vi "test_udp_write.vi"() -> ()   [LabVIEW 2019]
uses:
  <vilib>/Utility/tcp.llb/UDP Multicast Write-Only Open.vi
panel:
  in  "stop":bool
  out "error out":errorcluster
  in  "TopUDPPort":u16=17308
  in  "TopTCPPort":u16=17309
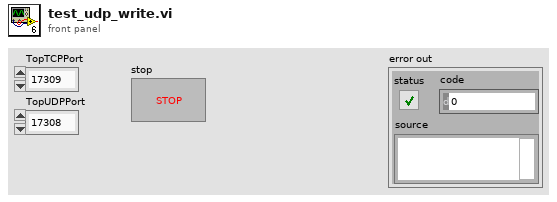
[diagram p1: front panel]
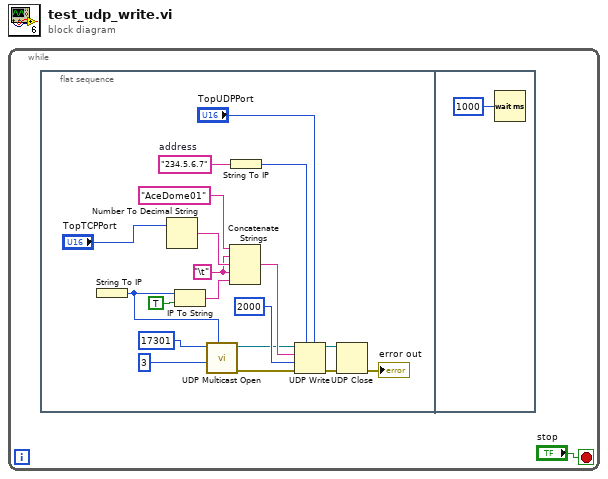
[diagram p0: block diagram]
diagram:
  n1 = while {
    stop <- "stop" stop-if-true
    n2 = flat-sequence {
      frame #0 {
        w13 = "\t"
        w18 = "234.5.6.7"  # address
        n3 = String To IP() -> (0:w6:u32)  [unwired: 1 in]
        n4 = Number To Decimal String(number="TopTCPPort") -> (decimal integer string=w15:string)  [unwired: 1 in]
        n5 = IP To String(1:TRUE ("dot notation? (F)"), 2:w6) -> (0:w11:string)
        n6 = call-poly <vilib>:"UDP Multicast Open.vi"("net address"=w6, "time-to-live (1)"=u16 3, "port"=u16 17301) -> ("error out"=w7:errorcluster, "connection ID"=w8:refnum<k16>)  [unwired: 7 in]
        n7 = Concatenate Strings("AceDome01" ("string"), w13, w15, w13, w11) -> (w10:string)
        n8 = String To IP(1:w18) -> (0:w17:u32)
        n9 = UDP Write(address=w17, port or service name="TopUDPPort", connection ID=w8, data in=w10, 8:w7, 9:2000 ("timeout ms (25000)")) -> (error out=w3:errorcluster, 3:w4:refnum<k16>)
        n10 = UDP Close(connection ID=w4, 8:w3) -> (error out=→"error out":errorcluster)  [unwired: 1 out]
      }
      frame #1 {
        n11 = Wait (ms)(milliseconds to wait=u32 1000) -> ()  [unwired: 1 out]
      }
    }
  }
